vi "RT.vi"() -> ()   [LabVIEW 2018]
uses:
  <vilib>/FPGAPlugInAG/sbRIO-9607/niLvFpga_Open_sbRIO-9607.vi
  <vilib>/rvi/interface/common/dynamic/niFpgaDynamicAddResources.vi
  <vilib>/Utility/error.llb/Error Cluster From Error Code.vi
  <vilib>/rvi/errors/niLvFpgaAdjustHostInterfaceError.vi
  <vilib>/FPGAPlugInAG/Dynamic/niLvFpga_Close_Dynamic.vi
  <vilib>/rvi/interface/nirviOpenFPGA/nirviOpenFPGA.xnode
  FPGA Bitfiles/SPIFast_FPGATarget_FPGA_ir-wfT85u8U.lvbitx
  FPGA.vi
  <vilib>/rvi/interface/nirviReadWriteControl/nirviReadWriteControl.xnode
  <vilib>/rvi/interface/nirviCloseFPGA/nirviCloseFPGA.xnode
  NiFpgaLv.dll
  <vilib>/rvi/interface/Simulation/niFpgaSimulationCallBeginRW.vi
panel:
  in  "SP 4":u16
  in  "SP 3":u16
  out "Byte 3":u16
  out "Byte 2":u16
  in  "dsPIC33":T1(ring)
  in  "SP 2":u16
  in  "SP":u16
  out "Byte 1":u16
  out "Byte 0":u16
  in  "Stop Button":bool
  in  "Pause":u8=20
  in  "Clock":u8=180
  in  "SPI":bool
  out "Error Out":errorcluster
  in  "Error In":errorcluster
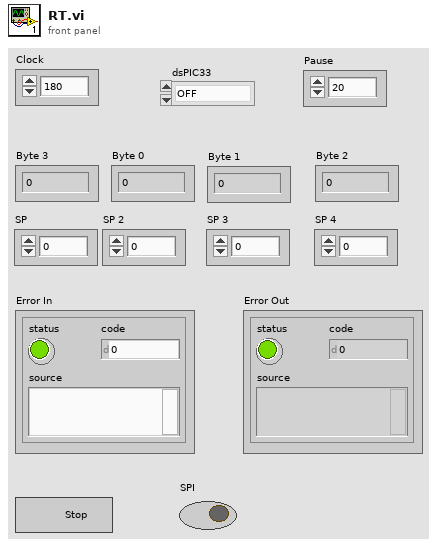
[diagram p1: front panel]
types:
  T1 = enum16{"OFF", "Voltage", "Curtain", "Corona", "Heater"}
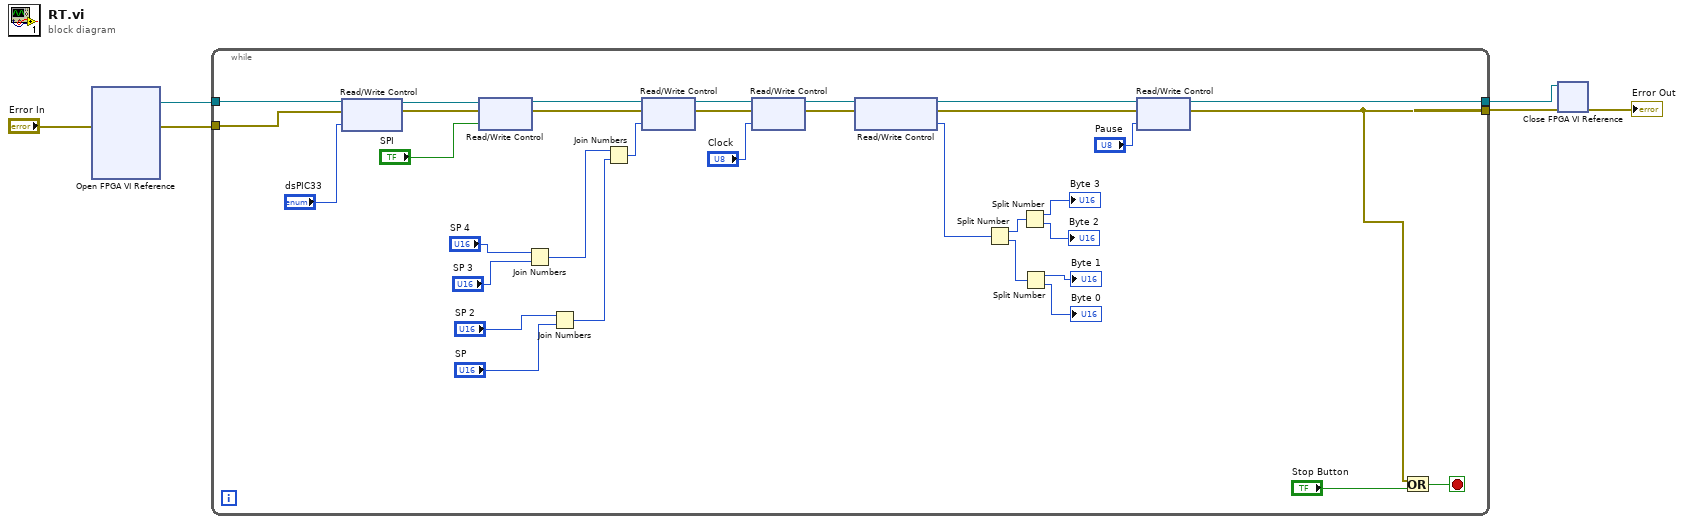
[diagram p0: block diagram]
diagram:
  n1 = xnode "Open FPGA VI Reference"("error in"="Error In") -> ("FPGA VI Reference Out"=w6:refnum<k20>, "error out"=w5:errorcluster)  [unwired: 1 in]
  n2 = while {
    tunnel: w6 -> [w34]
    tunnel: w5 -> [w29]
    tunnel: [w22] -> w2
    tunnel: [w23] -> w1
    stop <- w25 stop-if-true
    n3 = xnode "Read/Write Control"("FPGA VI Reference In"=w34, "error in"=w29, "dsPIC33"="dsPIC33") -> ("FPGA VI Reference Out"=w33:refnum<k20>, "error out"=w30:errorcluster)
    n4 = xnode "Read/Write Control"("FPGA VI Reference In"=w33, "error in"=w30, "Write"="SPI") -> ("FPGA VI Reference Out"=w32:refnum<k20>, "error out"=w31:errorcluster)
    n5 = Join Numbers(hi="SP 4", lo="SP 3") -> ((hi.lo)=w12:u32)
    n6 = Join Numbers(hi="SP 2", lo="SP") -> ((hi.lo)=w15:u32)
    n7 = Join Numbers(hi=w12, lo=w15) -> ((hi.lo)=w16:u64)
    n8 = xnode "Read/Write Control"("FPGA VI Reference In"=w32, "error in"=w31, "Data"=w16) -> ("FPGA VI Reference Out"=w37:refnum<k20>, "error out"=w38:errorcluster)
    n9 = xnode "Read/Write Control"("FPGA VI Reference In"=w37, "error in"=w38, "Delay"="Clock") -> ("FPGA VI Reference Out"=w39:refnum<k20>, "error out"=w40:errorcluster)
    n10 = xnode "Read/Write Control"("FPGA VI Reference In"=w39, "error in"=w40) -> ("FPGA VI Reference Out"=w27:refnum<k20>, "error out"=w28:errorcluster, "PIC Monitor"=w11:u64)
    n11 = Split Number(x=w11) -> (hi(x)=w9:u32, lo(x)=w10:u32)
    n12 = Split Number(x=w9) -> (hi(x)=→"Byte 3":u16, lo(x)=→"Byte 2":u16)
    n13 = Split Number(x=w10) -> (hi(x)=→"Byte 1":u16, lo(x)=→"Byte 0":u16)
    n14 = xnode "Read/Write Control"("FPGA VI Reference In"=w27, "error in"=w28, "Pause"="Pause") -> ("FPGA VI Reference Out"=w23:refnum<k20>, "error out"=w22:errorcluster)
    n15 = Or(x=w22, y="Stop Button") -> (x .or. y?=w25:bool)
  }
  n16 = xnode "Close FPGA VI Reference"("FPGA VI Reference In"=w1, "error in"=w2) -> ("error out"=→"Error Out":errorcluster)
